vi "Read Temperature.vi"(8 "error in (no error)":errorcluster, 11 "Gesture Sensor in":refnum<class "I2C Thermocouple.lvclass">) -> (0 "error out":errorcluster, 2 "Temperature":dbl, 3 "Gesture Sensor out":refnum<class "I2C Thermocouple.lvclass">)   [LabVIEW 2020, in "CTI-Peripheral.lvlib" / "I2C Thermocouple.lvclass"]
uses:
  I2C Thermocouple.lvclass
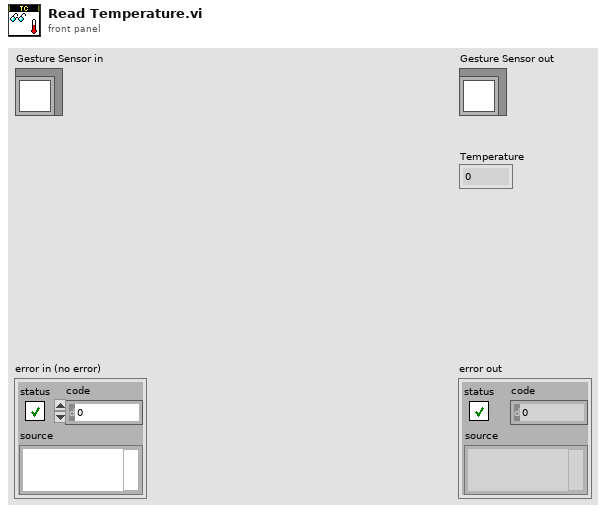
[diagram p1: front panel]
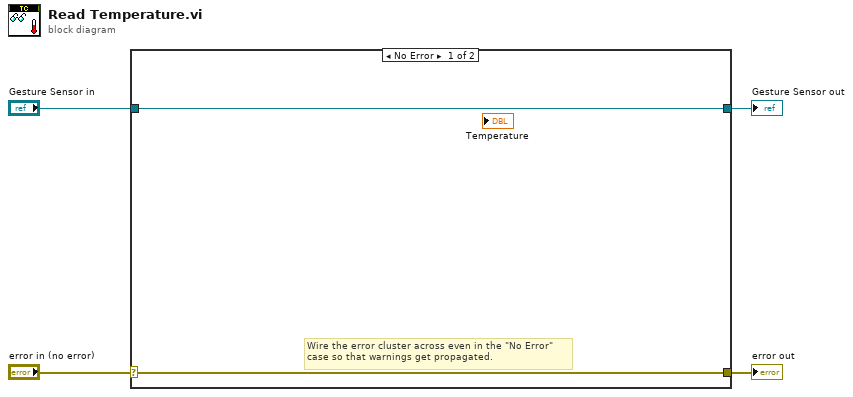
[diagram p0: block diagram]
diagram:
  n1 = case shown="No Error" "error in (no error)" {
    selector: "error in (no error)" -> [w5 w8]
    tunnel: [w5 w8] -> w3
    tunnel: [w6 w7] -> w1
    tunnel: "Gesture Sensor in" -> [w6 w7]
    frame No Error {
      # "Wire the error cluster across even in the \"No Error\"\ncase so that warnings get propagated."
    }
    frame Error {
    }
  }
  "error out" <- w3
  "Gesture Sensor out" <- w1
